vi "TESTE.vi"   [LabVIEW 2018]
uses:
  Simulated_CCD_Camera/Simulated Camera.lvclass
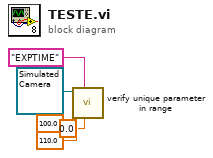
[diagram p0: block diagram]
diagram:
  n1 = call "verify unique parameter in range.vi"("lower limit"=0.0, "parameter name"="EXPTIME", "value"=110.0, "upper limit"=100.0, "Simulated_CCD_Camera in"=refnum<class "Simulated Camera.lvclass"> refnum) -> ()  [unwired: 5 in, 2 out]
